vi "Autosize.vi"(8 "error in":errorcluster, 11 "Philips Dialog in":refnum<class "Flex UI Dialog.lvclass">) -> (0 "error out":errorcluster, 3 "Philips Dialog out":refnum<class "Flex UI Dialog.lvclass">)   [LabVIEW 2014, in "Flex UI Dialog.lvclass"]
uses:
  Flex UI Dialog.lvclass
  Flex UI (Parent)/Flex UI.lvclass/Flex UI.ctl
  Flex UI (Parent)/Flex UI.lvclass
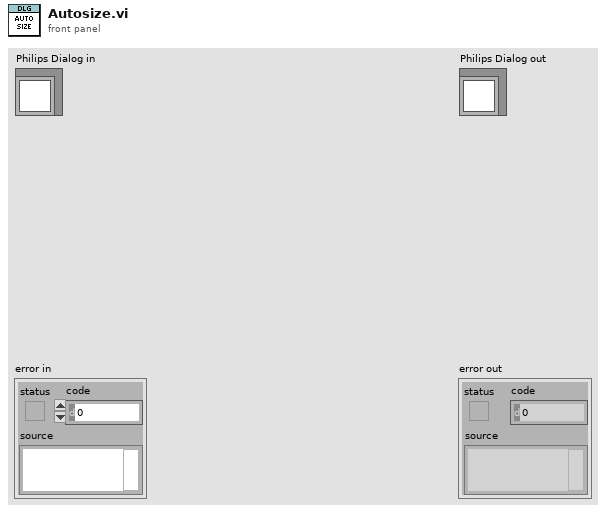
[diagram p1: front panel]
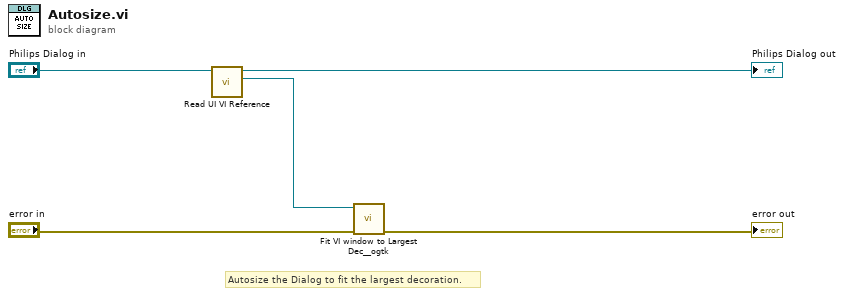
[diagram p0: block diagram]
diagram:
  # "Autosize the Dialog to fit the largest decoration."
  n1 = call "Read UI VI Reference.vi"("Philips UI in"="Philips Dialog in") -> ("UI VI Reference"=w1:refnum<vi>, "Philips UI out"=→"Philips Dialog out":refnum<class "Flex UI Dialog.lvclass">)  [unwired: 9 in]
  n2 = call <userlib>:"Fit VI window to Largest Dec__ogtk.vi"("error in (no error)"="error in", "VI Ref (calling VI)"=w1) -> ("error out"=→"error out":errorcluster)  [unwired: 4 in, 1 out]
